vi "Intan_filter_signals_for_display_v2.vi"(1 "Center Traces":bool, 2 "input filter cluster":T1={"LP Filter On/Off"=FALSE, "LP Cutoff (Hz)"=0.0, "HP Filter On/Off"=FALSE, "HP Cutoff (Hz)"=0.0, "Bandstop On/Off"=FALSE, "fl Cutoff (Hz)"=48.0, "fh Cutoff (Hz) "=52.0}, 3 "Sample Rate (Hz)":dbl, 4 "Nchan Array In [Nchans x Nsamps]":dbl[][](array[numeric])=array32x200[6400 elements]) -> (0 "Display Signals Out [Nchans x Nsamps]":dbl[][](array[numeric]))   [LabVIEW 2015]
uses:
  <vilib>/Analysis/3filter.llb/Filter Passband Type.ctl
  <vilib>/Analysis/3filter.llb/IIR Cascade Filter with I.C. (DBL).vi
  <vilib>/Analysis/NI_AALBase.lvlib
panel:
  out "LPF Final Filter State":dbl[][](array[numeric])
  out "HPF Final Filter State":dbl[][](array[numeric])
  out "BSF Filter State":dbl[][](array[numeric])
  out "First Call?: T/F":bool
  out "iter":i32
  out "Forloopiters":i32
  out "Nsamps":i32
  out "Nchans":i32
  out "chandata":dbl[](array[numeric])
  out "filt signal avg":dbl[](array[numeric])
  out "raw signal avg":dbl[](array[numeric])
  out "element subtracted":dbl
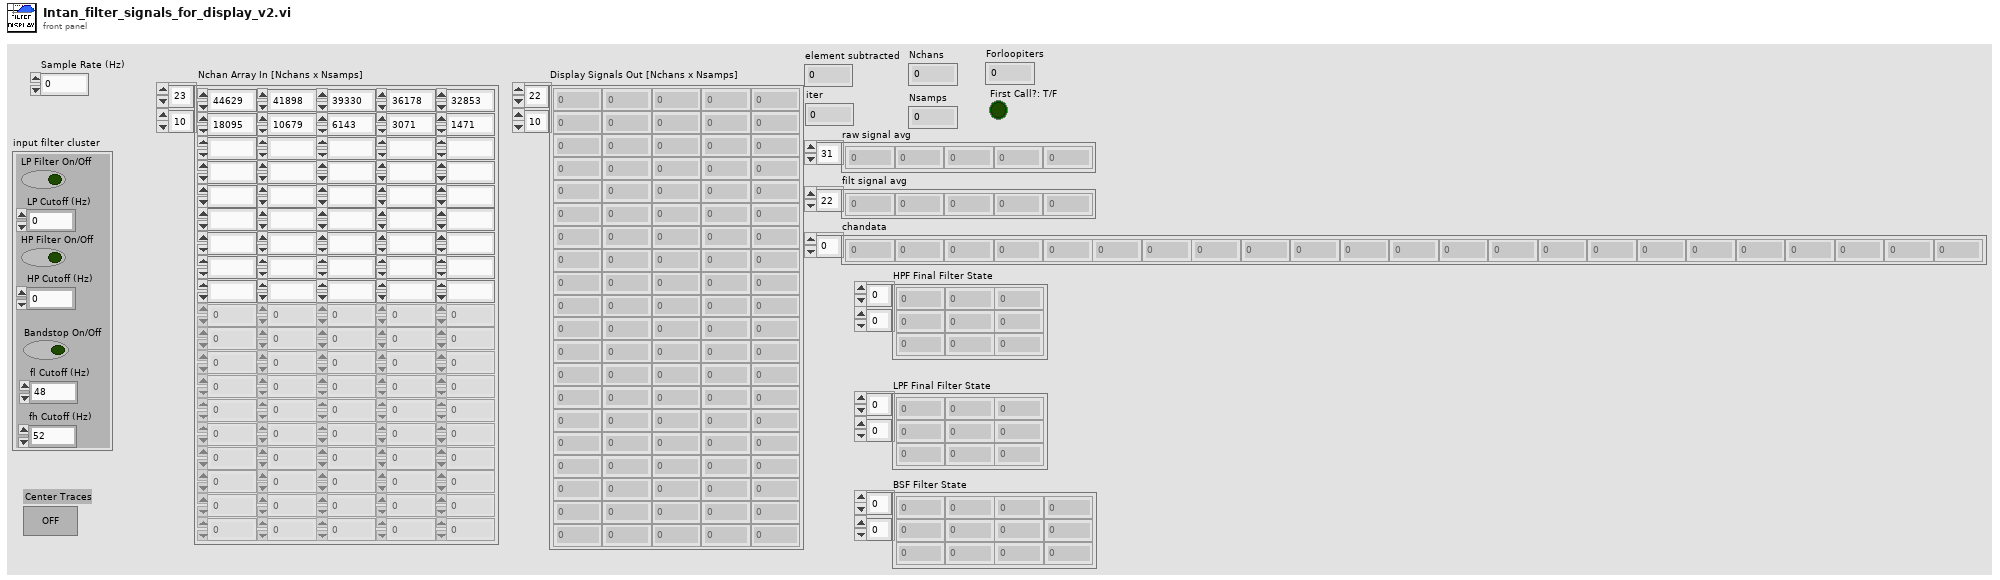
[diagram p1: front panel]
types:
  T1 = cluster{"LP Filter On/Off":bool, "LP Cutoff (Hz)":dbl, "HP Filter On/Off":bool, "HP Cutoff (Hz)":dbl, "Bandstop On/Off":bool, "fl Cutoff (Hz)":dbl, "fh Cutoff (Hz) ":dbl}
  T2 = typedef "NI_AALBase.lvlib/Filter Passband Type.ctl" = enum32{"Lowpass", "Highpass", "Bandpass", "Bandstop"}
  T3 = enum32{"Lowpass", "Highpass", "Bandpass", "Bandstop"}
  T4 = cluster{"filter structure":enum32{"IIR 2nd Order", "IIR 4th Order"}, "Reverse Coefficients":dbl[], "Forward Coefficients":dbl[]}
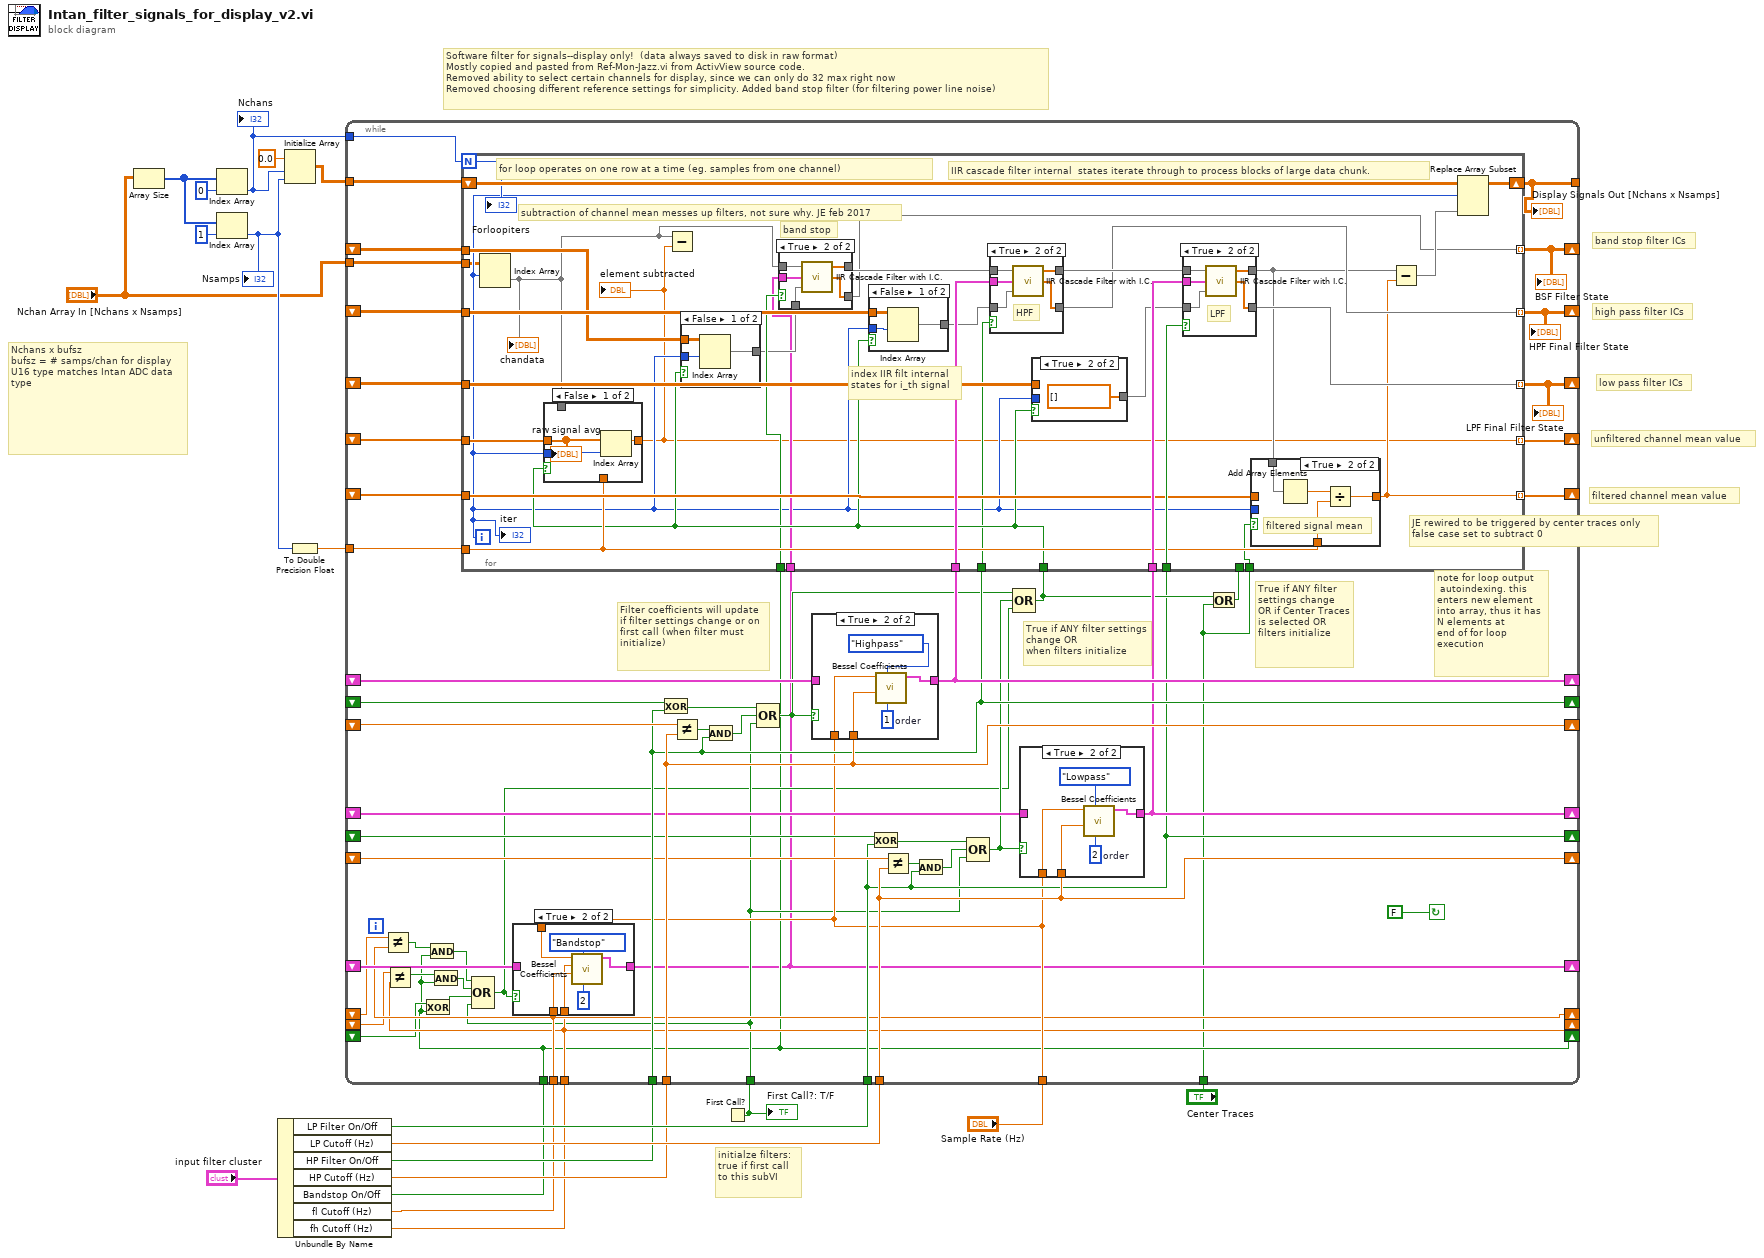
[diagram p0: block diagram]
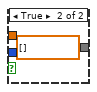
[diagram p5: hidden frame]
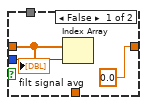
[diagram p7: hidden frame]
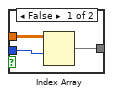
[diagram p8: hidden frame]
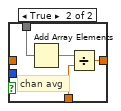
[diagram p9: hidden frame]
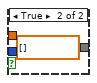
[diagram p12: hidden frame]
diagram:
  # "JE rewired to be triggered by center traces only\nfalse case set to subtract 0"
  # "filtered channel mean value"
  # "unfiltered channel mean value"
  # "low pass filter ICs"
  # "high pass filter ICs"
  # "band stop filter ICs"
  # "Nchans x bufsz \nbufsz = # samps/chan for display\nU16 type matches Intan ADC data type"
  # "Software filter for signals--display only!  (data always saved to disk in raw format)\nMostly copied and pasted from Ref-Mon-Jazz.vi from ActivView source code.\nRemoved ability to select certain channels for display, since we can only do 32 max right now\nRemoved choosing different reference settings for simplicity. Added band stop filter (for filtering power line noise)"
  # "initialze filters:\ntrue if first call\nto this subVI"
  n1 = Array Size(array="Nchan Array In [Nchans x Nsamps]") -> (size(s)=w13:i32[])
  n2 = Index Array(array=w13, index=0) -> (element=w2:i32)
  "Nchans" <- w2
  n3 = Index Array(array=w13, index=1) -> (element=w10:i32)
  "Nsamps" <- w10
  n4 = Unbundle By Name("input filter cluster") -> ("LP Filter On/Off"=w20:bool, "LP Cutoff (Hz)"=w18:dbl, "HP Filter On/Off"=w17:bool, "HP Cutoff (Hz)"=w16:dbl, "Bandstop On/Off"=w3:bool, "fl Cutoff (Hz)"=w5:dbl, "fh Cutoff (Hz)"=w4:dbl)
  n5 = Initialize Array(0.0 ("element"), w2, w10) -> (w14:dbl[][])
  n6 = To Double Precision Float(number=w10) -> (double precision float=w9:dbl)
  n7 = First Call?() -> (First Call?: T/F=w7:bool)
  "First Call?: T/F" <- w7
  n8 = while {
    shift-left: _ -> [w75]
    shift-right: [w74] -> _
    shift-right: [w67] -> _
    shift-left: _ -> [w68]
    shift-right: [w72] -> _
    shift-left: _ -> [w71]
    shift-right: [w69] -> _
    shift-left: _ -> [w70]
    tunnel: "Nchan Array In [Nchans x Nsamps]" -> [w66]
    tunnel: w9 -> [w65]
    shift-right: [w60] -> _
    shift-left: _ -> [w61]
    shift-right: [w56] -> _
    shift-left: _ -> [w59]
    shift-right: [w57] -> _
    shift-left: _ -> [w58]
    tunnel: w16 -> [w57]
    tunnel: w7 -> [w33]
    tunnel: "Sample Rate (Hz)" -> [w41]
    tunnel: w17 -> [w56]
    shift-right: [w51] -> _
    shift-left: _ -> [w52]
    shift-right: [w45] -> _
    shift-left: _ -> [w50]
    shift-right: [w48] -> _
    shift-left: _ -> [w49]
    tunnel: w18 -> [w48]
    tunnel: w20 -> [w45]
    tunnel: "Center Traces" -> [w23]
    tunnel: w14 -> [w42]
    tunnel: [w21] -> _
    tunnel: w5 -> [w39]
    tunnel: w4 -> [w37]
    tunnel: w3 -> [w27]
    shift-right: [w26] -> _
    shift-left: _ -> [w40]
    shift-right: [w37] -> _
    shift-left: _ -> [w36]
    shift-right: [w39] -> _
    shift-left: _ -> [w38]
    shift-right: [w27] -> _
    shift-left: _ -> [w35]
    shift-right: [w25] -> _
    shift-left: _ -> [w24]
    tunnel: w2 -> [w22]
    stop <- FALSE continue-if-true
    # "note for loop output\n autoindexing. this\nenters new element \ninto array, thus it has\nN elements at \nend of for loop\nexecution"
    # "True if ANY filter settings change\nOR if Center Traces is selected OR filters initialize"
    # "True if ANY filter settings change OR\nwhen filters initialize"
    # "Filter coefficients will update if filter settings change or on first call (when filter must initialize)"
    n9 = Not Equal?(x=w38, y=w39) -> (x != y?=w30:bool)
    n10 = Not Equal?(x=w36, y=w37) -> (x != y?=w29:bool)
    n11 = Exclusive Or(1:w27, 2:w35) -> (0:w34:bool)
    n12 = And(x=w30, y=w27) -> (x .and. y?=w31:bool)
    n13 = And(x=w29, y=w27) -> (x .and. y?=w32:bool)
    n14 = Compound Arithmetic op=OR(w31, w32, w34, w33) -> (w28:bool)
    n15 = case shown="True" w28 {
      tunnel: w39 -> [_ w80]
      tunnel: w37 -> [_ w79]
      tunnel: w41 -> [_ w78]
      tunnel: [w76 w77] -> w26
      tunnel: w40 -> [w76 _]
      frame False {
      }
      frame True {
        n16 = call <vilib>:"Bessel Coefficients.vi"("order"=2, "filter type"=Filter_Passband_Type."Bandstop", "low cutoff freq: fl"=w80, "high cutoff freq: fh"=w79, "sampling freq: fs"=w78) -> ("IIR Filter Cluster"=w77:T4)  [unwired: 5 in, 1 out]
      }
    }
    n17 = Exclusive Or(1:w56, 2:w59) -> (0:w64:bool)
    n18 = Not Equal?(x=w58, y=w57) -> (x != y?=w63:bool)
    n19 = And(x=w63, y=w56) -> (x .and. y?=w62:bool)
    n20 = Compound Arithmetic op=OR(w64, w62, w33) -> (w43:bool)
    n21 = case shown="True" w43 {
      tunnel: w57 -> [_ w91]
      tunnel: w41 -> [_ w93]
      tunnel: [w89 w94] -> w60
      tunnel: w61 -> [w89 _]
      frame False {
      }
      frame True {
        w92 = 1  # order
        n22 = call <vilib>:"Bessel Coefficients.vi"("order"=w92, "filter type"=T3."Highpass", "low cutoff freq: fl"=w91, "sampling freq: fs"=w93) -> ("IIR Filter Cluster"=w94:T4)  [unwired: 6 in, 1 out]
      }
    }
    n23 = Exclusive Or(1:w45, 2:w50) -> (0:w55:bool)
    n24 = Not Equal?(x=w49, y=w48) -> (x != y?=w54:bool)
    n25 = And(x=w54, y=w45) -> (x .and. y?=w53:bool)
    n26 = Compound Arithmetic op=OR(w55, w53, w33) -> (w44:bool)
    n27 = Compound Arithmetic op=OR(w43, w44, w28) -> (w46:bool)
    n28 = case shown="True" w44 {
      tunnel: w48 -> [_ w87]
      tunnel: w41 -> [_ w86]
      tunnel: [w83 w88] -> w51
      tunnel: w52 -> [w83 _]
      frame False {
      }
      frame True {
        w85 = 2  # order
        n29 = call <vilib>:"Bessel Coefficients.vi"("order"=w85, "filter type"=T3."Lowpass", "low cutoff freq: fl"=w87, "sampling freq: fs"=w86) -> ("IIR Filter Cluster"=w88:T4)  [unwired: 6 in, 1 out]
      }
    }
    n30 = Or(x=w46, y=w23) -> (x .or. y?=w47:bool)
    n31 = for {
      N: w22 -> [w100]
      tunnel: w75 -> [w118]
      tunnel: [w120] -> w74 mode=indexing
      tunnel: w60 -> [w126]
      tunnel: w46 -> [w108]
      tunnel: w56 -> [w106]
      tunnel: [w123] -> w72 mode=indexing
      tunnel: w71 -> [w117]
      tunnel: w51 -> [w122]
      tunnel: w45 -> [w121]
      tunnel: w70 -> [w114]
      tunnel: [w113] -> w69 mode=indexing
      tunnel: w47 -> [_]
      tunnel: w68 -> [w119]
      tunnel: [w96] -> w67 mode=indexing
      tunnel: w66 -> [w98]
      tunnel: w65 -> [w109]
      shift-right: [w110] -> w21
      shift-left: w42 -> [w112]
      tunnel: w27 -> [w105]
      tunnel: w26 -> [w103]
      tunnel: [w102] -> w25 mode=indexing
      tunnel: w24 -> [w101]
      tunnel: w23 -> [w97]
      i -> [w99]
      # "subtraction of channel mean messes up filters, not sure why. JE feb 2017"
      # "band stop"
      # "index IIR filt internal states for i_th signal"
      # "IIR cascade filter internal  states iterate through to process blocks of large data chunk."
      # "for loop operates on one row at a time (eg. samples from one channel)"
      n32 = Index Array(array=w98, index (row)=w99) -> (element=w95:dbl[])  [unwired: 1 in]
      "chandata" <- w95
      n33 = case shown="False" w108 {
        tunnel: w95 -> [_ w154]
        tunnel: [w149 w153] -> w96
        tunnel: w119 -> [w151 _]
        tunnel: w99 -> [w150 _]
        tunnel: w109 -> [_ w152]
        frame False {
          n34 = Index Array(array=w151, index=w150) -> (element=w149:dbl)
          "raw signal avg" <- w151
        }
        frame True {
          # "chan avg"
          n35 = Add Array Elements(numeric array=w154) -> (sum=w155:dbl)
          n36 = Divide(x=w155, y=w152) -> (x/y=w153:dbl)
        }
      }
      "element subtracted" <- w96
      n37 = Subtract(x=w95, y=w96) -> ()  [unwired: 1 out]
      n38 = case shown="False" w108 {
        tunnel: [w127 dbl[] [] ("Initial Filter State")] -> w104
        tunnel: w101 -> [w129 _]
        tunnel: w99 -> [w128 _]
        frame False {
          n39 = Index Array(array=w129, index (row)=w128) -> (element=w127:dbl[])  [unwired: 1 in]
        }
        frame True {
        }
      }
      n40 = case shown="True" w105 {
        tunnel: [w131 w137] -> w102
        tunnel: [w132 w136] -> w107
        tunnel: w95 -> [w132 w135]
        tunnel: w104 -> [w131 w134]
        tunnel: w103 -> [_ w133]
        frame False {
        }
        frame True {
          n41 = call-poly <vilib>:"IIR Cascade Filter with I.C..vi"("Initial Filter State"=w134, "IIR Filter Cluster"=w133, "X"=w135) -> ("Final Filter State"=w137:dbl[], "Filtered X"=w136:dbl[])  [unwired: 1 out]
        }
      }
      n42 = case shown="False" w108 {
        tunnel: [w170 dbl[] [] ("Initial Filter State")] -> w125
        tunnel: w118 -> [w172 _]
        tunnel: w99 -> [w171 _]
        frame False {
          n43 = Index Array(array=w172, index (row)=w171) -> (element=w170:dbl[])  [unwired: 1 in]
        }
        frame True {
        }
      }
      n44 = case shown="True" w106 {
        tunnel: w126 -> [_ w169]
        tunnel: [w163 w168] -> w120
        tunnel: w125 -> [w163 w165]
        tunnel: [w164 w167] -> w124
        tunnel: w107 -> [w164 w166]
        frame False {
        }
        frame True {
          # "HPF"
          n45 = call-poly <vilib>:"IIR Cascade Filter with I.C..vi"("Initial Filter State"=w165, "IIR Filter Cluster"=w169, "X"=w166) -> ("Final Filter State"=w168:dbl[], "Filtered X"=w167:dbl[])  [unwired: 1 out]
        }
      }
      n46 = case shown="True" w108 {
        tunnel: [w145 dbl[] [] ("Initial Filter State")] -> w116
        tunnel: w117 -> [w147 _]
        tunnel: w99 -> [w146 _]
        frame False {
          n47 = Index Array(array=w147, index (row)=w146) -> (element=w145:dbl[])  [unwired: 1 in]
        }
        frame True {
        }
      }
      n48 = case shown="True" w121 {
        tunnel: w122 -> [_ w162]
        tunnel: [w156 w161] -> w123
        tunnel: w116 -> [w156 w160]
        tunnel: [w157 w159] -> w115
        tunnel: w124 -> [w157 w158]
        frame False {
        }
        frame True {
          # "LPF"
          n49 = call-poly <vilib>:"IIR Cascade Filter with I.C..vi"("Initial Filter State"=w160, "IIR Filter Cluster"=w162, "X"=w158) -> ("Final Filter State"=w161:dbl[], "Filtered X"=w159:dbl[])  [unwired: 1 out]
        }
      }
      n50 = case shown="True" w97 {
        tunnel: w115 -> [_ w142]
        tunnel: [0.0 w144] -> w113
        tunnel: w114 -> [w140 _]
        tunnel: w99 -> [w139 _]
        tunnel: w109 -> [_ w141]
        frame False {
          n51 = Index Array(array=w140, index=w139) -> ()  [unwired: 1 out]
          "filt signal avg" <- w140
        }
        frame True {
          # "filtered signal mean"
          n52 = Add Array Elements(numeric array=w142) -> (sum=w143:dbl)
          n53 = Divide(x=w143, y=w141) -> (x/y=w144:dbl)
        }
      }
      n54 = Subtract(x=w115, y=w113) -> (x-y=w111:dbl[])
      n55 = Replace Array Subset(array=w112, new element=w111, index (row)=w99) -> (w110:dbl[][])  [unwired: 1 in]
      "Forloopiters" <- w100
      "iter" <- w99
    }
    "BSF Filter State" <- w25
    "HPF Final Filter State" <- w74
    "LPF Final Filter State" <- w72
    "Display Signals Out [Nchans x Nsamps]" <- w21
  }
